vi "SerialMultiplex.vi"(1 "FlowMeter":refnum<k21>="Mod6\\Port1", 2 "PumpVFD":refnum<k21>="Mod6\\Port1") -> ()   [LabVIEW 2023]
uses:
  <vilib>/rvi/Emulation/niFpgaGetClockAttributes.vi
  <vilib>/rvi/Emulation/niFpgaSctlEmulationGetInTimedLoop.vi
  <vilib>/rvi/Emulation/niFpgaEmulationReportErrorSimple.vi
  <vilib>/rvi/DataTransferAndStorage/Container/Common/niFpgaContainerGetUniqueNameForEmu.vi
  <vilib>/rvi/DataTransferAndStorage/Container/Common/niFpgaContainerSetEmuInfo.vi
  <vilib>/rvi/eio/common/nirviEmuReportErrorAndStop.vi
  <vilib>/rvi/DataTransferAndStorage/Container/Common/niFpgaContainerExecOnDevCompGetState.vi
  <vilib>/rvi/Emulation/niFpgaEmulationIsFPGAContextNoSignature.vi
  <vilib>/rvi/errors/niFpgaSetErrorForExecOnDevCompSimple.vi
  <vilib>/rvi/FIFO/Fifo_Resource/nirvififoEmulationSetSize.vi
  <vilib>/rvi/FIFO/Fifo_Resource/nirviFifoEmulationQueueMgr.vi
  <instcachedir>/0/nirviFifoEmulationQueueMgr_E5CAEC123FF24DC58D834DCA3CDAA9B5.lvgen/nirviFifoEmulationQueueMgr_E5CAEC123FF24DC58D834DCA3CDAA9B5_002.vi
  <vilib>/rvi/FIFO/Fifo_Resource/nirvififoEmulationDetermineInputValidOut.vi
  <vilib>/rvi/FIFO/Fifo_Resource/nirvififoEmulationCreateLock.vi
  <vilib>/rvi/Emulation/niFpgaProcessEmulError.vi
  <vilib>/rvi/FIFO/Fifo_Resource/nirvififoEmulationObtainLock.vi
  <vilib>/rvi/FIFO/Fifo_Resource/nirvififoEmulationReleaseLock.vi
  <vilib>/rvi/occurrence/nirviWaitOnOccurrenceBase.vi
  <vilib>/rvi/errors/nirviReportUnexpectedCaseInternalError.vi
  <vilib>/rvi/errors/nirviReportUnexpectedCaseInternalError (U32).vi
  <vilib>/Utility/error.llb/Clear Errors.vi
  <vilib>/eio/utilities/niEioResolveVilibRelativePath.vi
  <vilib>/rvi/interface/RandomDataEmulation/niFpgaRandomDataHandleErrors.vi
  <vilib>/rvi/Emulation/niFpgaCriticalErrorInLSC.vi
  <vilib>/rvi/LocalResourceManager/LocalResourceManager.xnode
  <vilib>/rvi/DataTransferAndStorage/Container/XNode/niFpgaContainer.xnode
  <vilib>/rvi/FIFO/Fifo_Resource/niFpgaFifoEmulationRefIn.vi
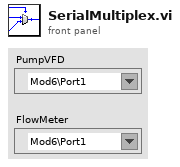
[diagram p1: front panel]
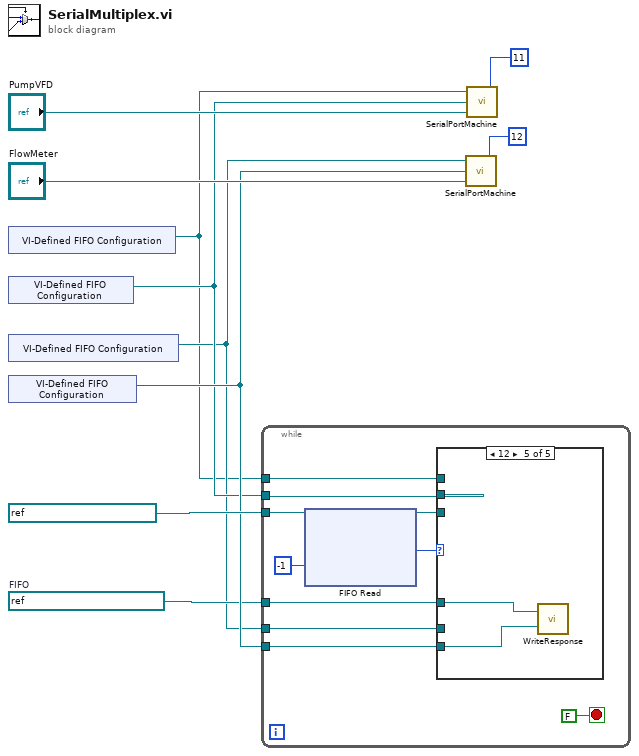
[diagram p0: block diagram]
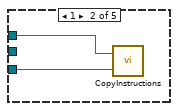
[diagram p3: hidden frame]
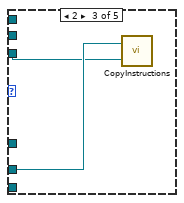
[diagram p4: hidden frame]
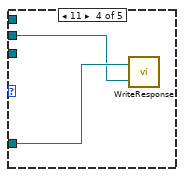
[diagram p5: hidden frame]
diagram:
  w5 = refnum<k21> "SerialMultiplexResponse"  # FIFO
  n1 = xnode "VI-Defined FIFO Configuration"() -> ("FIFO Out"=w3:refnum<k21>)
  n2 = xnode "VI-Defined FIFO Configuration"() -> ("FIFO Out"=w6:refnum<k21>)
  n3 = xnode "VI-Defined FIFO Configuration"() -> ("FIFO Out"=w4:refnum<k21>)
  n4 = xnode "VI-Defined FIFO Configuration"() -> ("FIFO Out"=w7:refnum<k21>)
  n5 = while {
    tunnel: refnum<k21> "SerialMultiplexRequest" ("Requests") -> [w20]
    tunnel: w3 -> [w17]
    tunnel: w6 -> [w13]
    tunnel: w7 -> [w14]
    tunnel: w5 -> [w12]
    tunnel: w4 -> [w11]
    stop <- FALSE stop-if-true
    n6 = xnode ("FIFO Read")("Timeout"=-1, "FIFO In"=w20) -> ("Element"=w18:u8, "FIFO Out"=w16:refnum<k21>)  [unwired: 1 out]
    n7 = case shown="12" w18 {
      tunnel: w17 -> [_ w22 _ _ _]
      tunnel: w16 -> [_ w21 w23 _ _]
      tunnel: w13 -> [_ _ _ w25 _]
      tunnel: w14 -> [_ _ _ _ w28]
      tunnel: w12 -> [_ _ _ w26 w27]
      tunnel: w11 -> [_ _ w24 _ _]
      frame 0, Default {
      }
      frame 1 {
        n8 = call "CopyInstructions.vi"("Instructions"=w21, "Copy"=w22) -> ()  [unwired: 1 in]
      }
      frame 2 {
        n9 = call "CopyInstructions.vi"("Instructions"=w23, "Copy"=w24) -> ()  [unwired: 1 in]
      }
      frame 11 {
        n10 = call "WriteResponse.vi"("Refnum in"=w25, "Out"=w26) -> ()  [unwired: 1 in]
      }
      frame 12 {
        n11 = call "WriteResponse.vi"("Refnum in"=w28, "Out"=w27) -> ()  [unwired: 1 in]
      }
    }
  }
  n12 = call "SerialPortMachine.vi"("IRQ Number"=u8 12, "Port"="FlowMeter", "FIFOout"=w7, "Instructions"=w4) -> ()  [unwired: 2 in]
  n13 = call "SerialPortMachine.vi"("IRQ Number"=u8 11, "Port"="PumpVFD", "FIFOout"=w6, "Instructions"=w3) -> ()  [unwired: 2 in]
